vi "Set Default Value.vi"(9 "Default C++ Value":string, 10 "Control Ref":refnum<vi>, 11 "String Writer in":refnum<class "String Writer.lvclass">) -> (1 "LabVIEW Default String":string, 2 "Control Ref Dup":refnum<vi>, 3 "String Writer out":refnum<class "String Writer.lvclass">)   [LabVIEW 2014, in "String Writer.lvclass"]
doc: "Copyright (c) 2016 Sze Howe Koh\n\nThis Source Code Form is subject to the terms of the Mozilla Public License, v. 2.0. If a copy of the MPL was not distributed with this file, You can obtain one at http://mozilla.org/MPL/2.0/."
uses:
  String Writer.lvclass
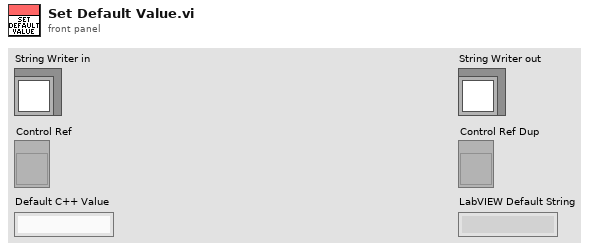
[diagram p1: front panel]
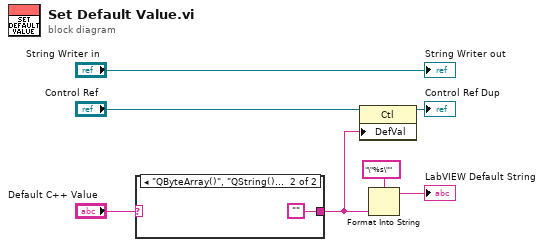
[diagram p0: block diagram]
diagram:
  n1 = case shown="\"QByteArray()\", \"QString()\"" "Default C++ Value" {
    selector: "Default C++ Value" -> [w8 _]
    tunnel: [w8 ""] -> w2
    frame Default {
    }
    frame "QByteArray()", "QString()" {
    }
  }
  n2 = property class="Ctl"(reference="Control Ref", "DefVal"=w2) -> (reference out=→"Control Ref Dup":refnum<vi>)  [unwired: 1 in, 1 out]
  n3 = Format Into String(format string="\"%s\"", w2) -> (resulting string=→"LabVIEW Default String":string)  [unwired: 2 in, 1 out]
  "String Writer out" <- "String Writer in"
